vi "upAndDown (SubVI).vi"(1 "Numeric":dbl) -> (0 "Numeric 2":dbl)   [LabVIEW 2019]
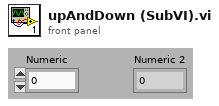
[diagram p1: front panel]
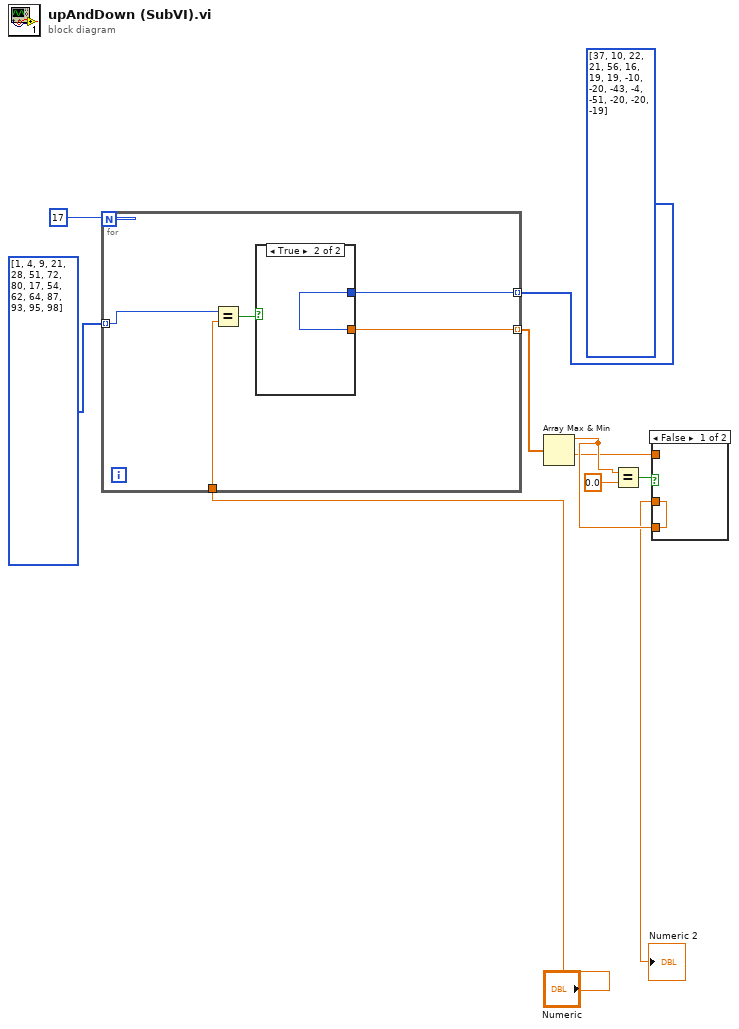
[diagram p0: block diagram]
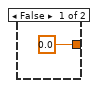
[diagram p3: hidden frame]
diagram:
  n1 = for {
    N: 17 -> [_]
    tunnel: i32[] [1, 4, 9, 21, 28, 51, 72, 80, 17, 54, 62, 64, 87, 93, 95, 98] -> [w13] mode=indexing
    tunnel: i32[] [37, 10, 22, 21, 56, 16, 19, 19, -10, -20, -43, -4, -51, -20, -20, -19] -> [w14] mode=indexing
    tunnel: "Numeric" -> [w12]
    tunnel: [w11] -> w3 mode=indexing
    n2 = Equal?(x=w13, y=w12) -> (x = y?=w15:bool)
    n3 = case shown="True" w15 {
      tunnel: [0.0 ("x") w17] -> w11
      tunnel: w14 -> [_ w17]
      frame False {
      }
      frame True {
      }
    }
  }
  n4 = Array Max & Min(array=w3) -> (max value=w8:dbl, min value=w7:dbl)  [unwired: 2 out]
  n5 = Equal?(x=w8, y=0.0) -> (x = y?=w4:bool)
  n6 = case shown="False" w4 {
    tunnel: [w18 w19] -> w6
    tunnel: w7 -> [_ w19]
    tunnel: w8 -> [w18 _]
    frame False {
    }
    frame True {
    }
  }
  "Numeric 2" <- w6
